vi "test_libssh2_sftp_statvfs.vi"() -> ()   [LabVIEW 2013, in "libssh2_integration_tests.lvlib"]
uses:
  libssh2_integration_tests.lvlib
  <vilib>/addons/_JKI Toolkits/Caraya/classes/Test/Test.lvclass
  libssh2/libssh2.lvlib
  <vilib>/addons/_JKI Toolkits/Caraya/classes/Assert/Assert.lvclass
panel:
  out "error out":errorcluster
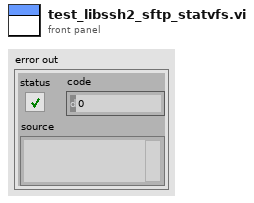
[diagram p1: front panel]
types:
  T1 = typedef "libssh2.lvlib/Session Refnum.ctl" = refnum<k1>
  T2 = typedef "libssh2.lvlib/SFTP Refnum.ctl" = refnum<k1>
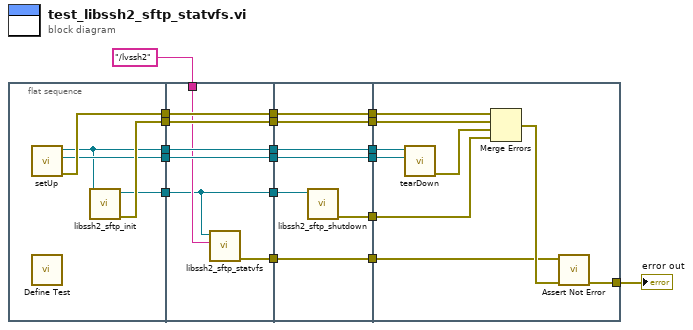
[diagram p0: block diagram]
diagram:
  n1 = flat-sequence {
    tunnel: [w24] -> w11
    tunnel: [w23] -> w10
    tunnel: [w22] -> w9
    tunnel: [w21] -> w8
    tunnel: [w20] -> w7
    tunnel: w11 -> [w31]
    tunnel: [w31] -> w6
    tunnel: w10 -> [w30]
    tunnel: [w30] -> w5
    tunnel: w9 -> [w26]
    tunnel: [w26] -> w4
    tunnel: w8 -> [w29]
    tunnel: [w29] -> w3
    tunnel: w7 -> [w28]
    tunnel: [w28] -> w2
    tunnel: "/lvssh2" ("filename") -> [w27]
    tunnel: [w25] -> w1
    tunnel: w2 -> [w38]
    tunnel: [w38] -> w18
    tunnel: w3 -> [w37]
    tunnel: [w37] -> w17
    tunnel: w4 -> [w34]
    tunnel: w5 -> [w36]
    tunnel: [w36] -> w16
    tunnel: w6 -> [w35]
    tunnel: [w35] -> w15
    tunnel: [w33] -> w14
    tunnel: w1 -> [w32]
    tunnel: [w32] -> w12
    tunnel: w18 -> [w47]
    tunnel: w17 -> [w46]
    tunnel: w16 -> [w45]
    tunnel: [w40] -> w19
    tunnel: w15 -> [w42]
    tunnel: w14 -> [w41]
    tunnel: w12 -> [w39]
    frame #0 {
      n2 = call "setUp.vi"() -> ("error out"=w23:errorcluster, "connection ID"=w21:refnum<k5>, "session"=w20:T1)  [unwired: 9 in]
      n3 = call <vilib>:"Define Test.vi"() -> ()  [unwired: 10 in, 2 out]
      n4 = call "libssh2_sftp_init.vi"("session"=w20) -> ("error out"=w24:errorcluster, "sftp"=w22:T2)  [unwired: 9 in]
    }
    frame #1 {
      n5 = call "libssh2_sftp_statvfs.vi"("path"=w27, "sftp"=w26) -> ("error out"=w25:errorcluster)  [unwired: 8 in, 1 out]
    }
    frame #2 {
      n6 = call "libssh2_sftp_shutdown.vi"("sftp"=w34) -> ("error out"=w33:errorcluster)  [unwired: 10 in]
    }
    frame #3 {
      n7 = call "tearDown.vi"("connection ID"=w46, "session"=w47) -> ("error out"=w44:errorcluster)  [unwired: 9 in]
      n8 = Merge Errors(w45, w42, w44, w41) -> (w43:errorcluster)
      n9 = call <vilib>:"Assert Not Error.vi"("error in (no error)"=w43, "Not Error?"=w39) -> ("error out"=w40:errorcluster)  [unwired: 8 in, 1 out]
    }
  }
  "error out" <- w19
